vi "CheckOnIdle.vi"(6 "DataMessageQueue":refnum<queue>, 7 "ClassQueue":refnum<queue>, 8 "error in (no error)":errorcluster, 9 "Timeout (5s)":dbl=5.0 min=0.0 max=10.0, 10 "ChangeOccured? (F)":bool, 11 "SensorBase in":refnum<class "SensorBase.lvclass">) -> (0 "Error Out":errorcluster, 2 "Wrote?":bool, 3 "SensorBase out":refnum<class "SensorBase.lvclass">)   [LabVIEW 2018, in "SensorPlugins.lvlib"]
doc: "This VI checks to see if the module's acquistion loop is in idle. If it is it updates the Class Typedefinition that is stored in the queue. If it is not it sends a message to place it in idle, checks again and then updates the type definition if it is."
uses:
  SensorPlugins.lvlib
  SensorBaseClass/SensorBase.lvclass
  clMessage.ctl
  CheckOnIdle.ctl
  <vilib>/Utility/error.llb/Error Cluster From Error Code.vi
  <vilib>/ErrorRing/Error Ring.xnode
panel:
  out "Restart":bool
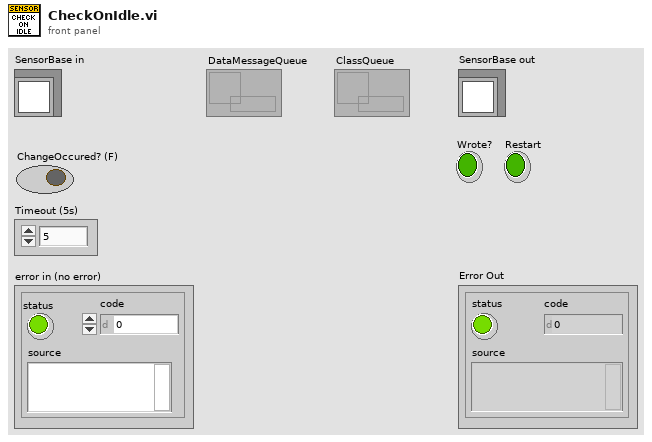
[diagram p1: front panel]
types:
  T1 = typedef "SensorPlugins.lvlib/CheckOnIdle.ctl" = enum16{"CheckOnState", "WriteToClassAndExit", "InIdle", "SetToStop", "Error", "Exit", "ReturnToStart"}
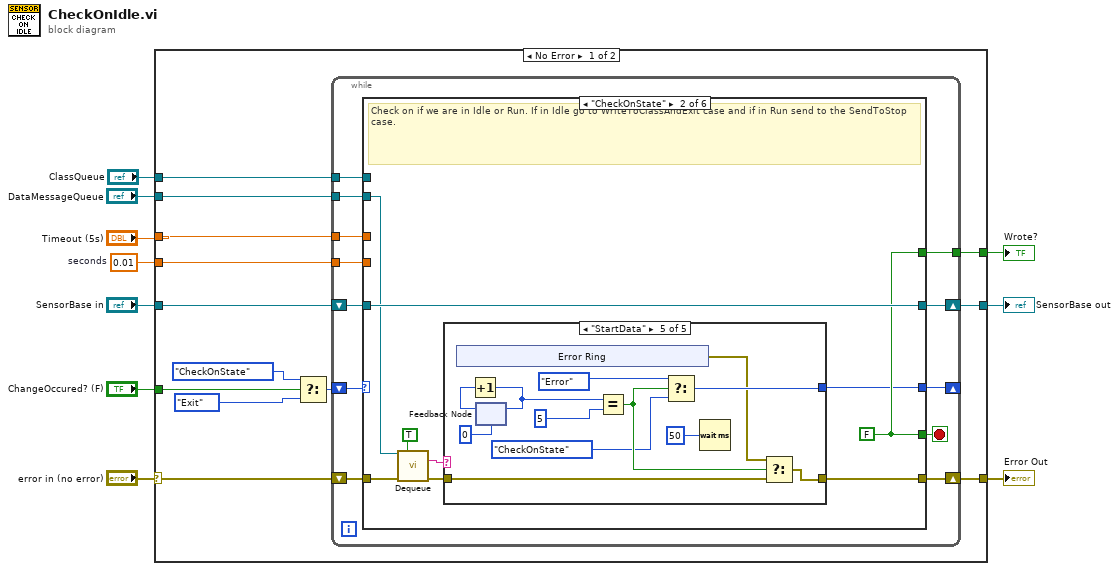
[diagram p0: block diagram]
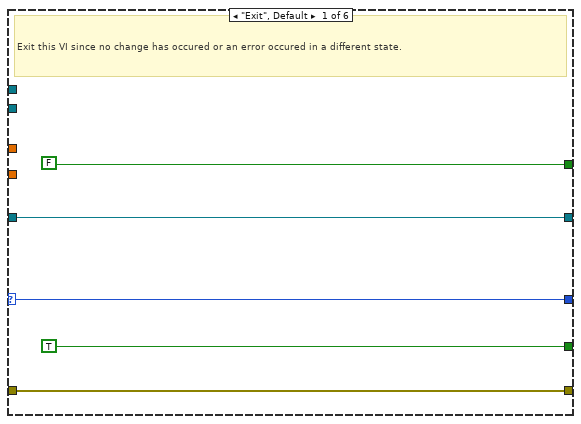
[diagram p2: hidden frame]
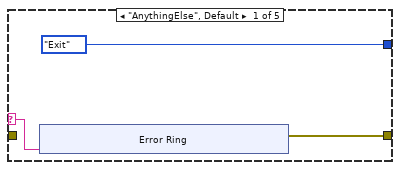
[diagram p3: hidden frame]
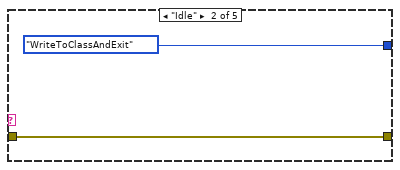
[diagram p4: hidden frame]
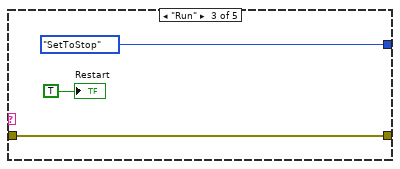
[diagram p5: hidden frame]
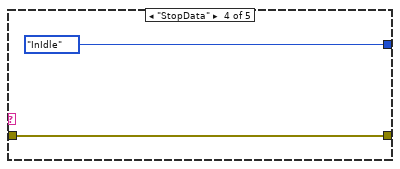
[diagram p6: hidden frame]
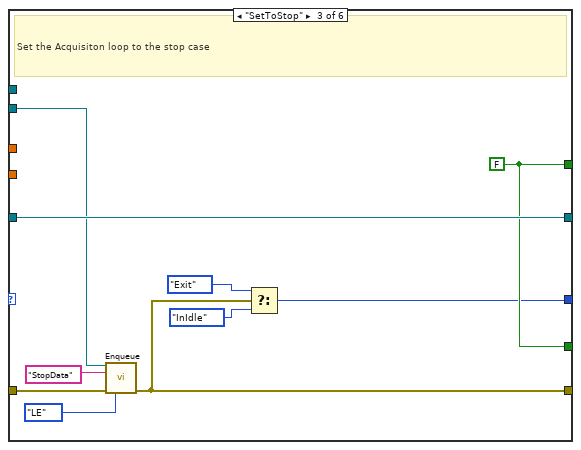
[diagram p7: hidden frame]
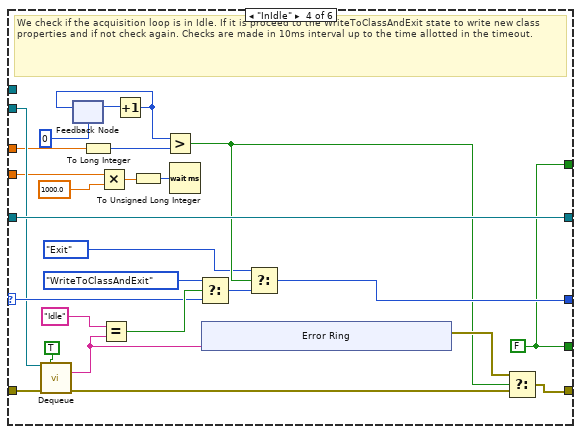
[diagram p8: hidden frame]
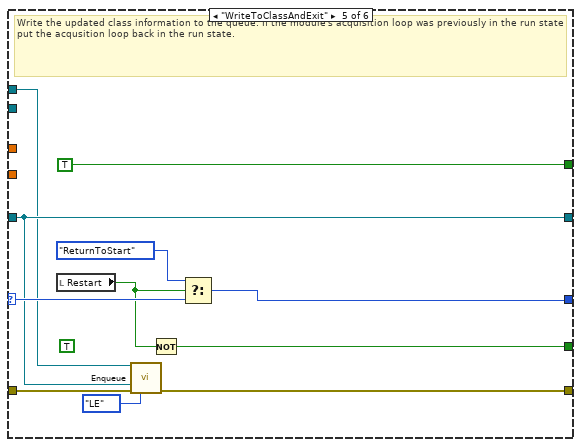
[diagram p9: hidden frame]
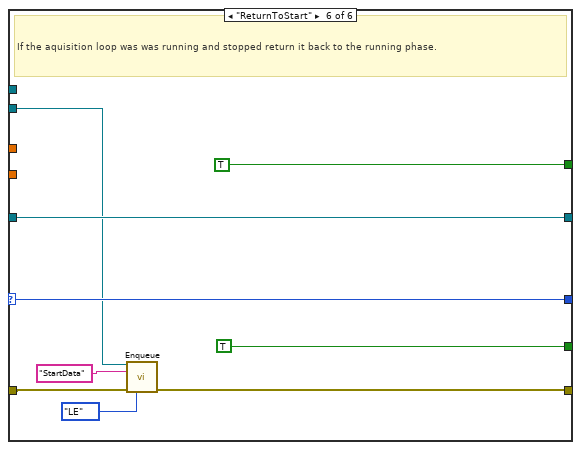
[diagram p10: hidden frame]
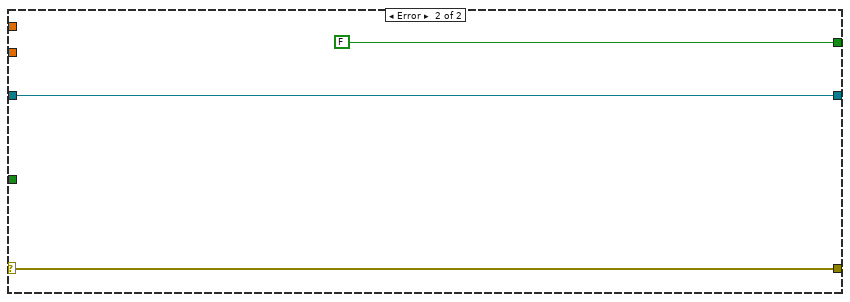
[diagram p11: hidden frame]
diagram:
  w9 = 0.01  # seconds
  n1 = case shown="No Error" "error in (no error)" {
    selector: "error in (no error)" -> [w22 w149]
    tunnel: "ChangeOccured? (F)" -> [w21 _]
    tunnel: "SensorBase in" -> [w20 w148]
    tunnel: [w19 w149] -> w6
    tunnel: "Timeout (5s)" -> [w18 _]
    tunnel: [w17 w148] -> w3
    tunnel: [w16 FALSE ("Set? (f)")] -> w5
    tunnel: "DataMessageQueue" -> [w15 _]
    tunnel: w9 -> [w14 _]
    tunnel: "ClassQueue" -> [w11 _]
    frame No Error {
      n2 = Select(t=CheckOnIdle."CheckOnState" ("Enum"), s=w21, f=CheckOnIdle."Exit" ("Enum")) -> (s? t:f=w23:T1)
      n3 = while {
        shift-right: [w30] -> _
        shift-left: w23 -> [w35]
        shift-right: [w32] -> w17
        shift-left: w20 -> [w33]
        shift-right: [w31] -> w19
        shift-left: w22 -> [w34]
        tunnel: w18 -> [w28]
        tunnel: [w27] -> w16
        tunnel: w15 -> [w26]
        tunnel: w14 -> [w25]
        tunnel: w11 -> [w24]
        stop <- w29 stop-if-true
        n4 = case shown="\"CheckOnState\"" w35 {
          selector: w35 -> [w39 _ _ w118 w134 w145]
          tunnel: w34 -> [w40 w48 w91 w111 w137 w140]
          tunnel: w33 -> [w38 w49 w93 w117 w128 w143]
          tunnel: [w40 w41 w88 w102 w130 w139] -> w31
          tunnel: [w38 w49 w93 w117 w128 w143] -> w32
          tunnel: [w39 w43 w87 w112 w135 w145] -> w30
          tunnel: [TRUE w45 w92 w104 w131 TRUE] -> w29
          tunnel: w28 -> [_ _ _ w96 _ _]
          tunnel: [FALSE ("Set? (f)") w45 w92 w104 TRUE ("Set? (f)") TRUE ("Set? (f)")] -> w27
          tunnel: w26 -> [_ w47 w90 w110 _ w138]
          tunnel: w25 -> [_ _ _ w106 _ _]
          tunnel: w24 -> [_ _ _ _ w127 _]
          frame "Exit", Default {
            # "Exit this VI since no change has occured or an error occured in a different state."
          }
          frame "CheckOnState" {
            w45 = FALSE
            # "Check on if we are in Idle or Run. If in Idle go to WriteToClassAndExit case and if in Run send to the SendToStop case."
            n5 = call "Dequeue.vi"("MessageQueue"=w47, "Preview Queue (F)"=TRUE ("PreviewQueue(F)"), "error in (no error)"=w48) -> ("Message"=w44:string, "error out"=w42:errorcluster)  [unwired: 8 in, 3 out]
            n6 = case shown="\"StartData\"" w44 {
              selector: w44 -> [w51 _ _ _ _]
              tunnel: [CheckOnIdle."Exit" ("Enum") CheckOnIdle."WriteToClassAndExit" ("Enum") CheckOnIdle."SetToStop" ("Enum") CheckOnIdle."InIdle" ("Enum") w76] -> w43
              tunnel: w42 -> [_ w61 w64 w66 w75]
              tunnel: [w52 w61 w64 w66 w74] -> w41
              frame "AnythingElse", Default {
                n7 = xnode "Error Ring"("parameter 0"=w51) -> ("error out"=w52:errorcluster)
              }
              frame "Idle" {
              }
              frame "Run" {
                "Restart" <- TRUE ("Restart")
              }
              frame "StopData" {
              }
              frame "StartData" {
                n8 = xnode "Error Ring"() -> ("error out"=w70:errorcluster)
                n9 = feedback #1(0) -> (w77:i32)
                n10 = Increment(x=w77) -> (x+1=w73:i32)
                n11 = feedback-in #1(w73) -> ()
                n12 = Equal?(x=w73, y=5 ("x")) -> (x = y?=w71:bool)
                n13 = Select(t=CheckOnIdle."Error" ("Enum"), s=w71, f=CheckOnIdle."CheckOnState" ("Enum")) -> (s? t:f=w76:T1)
                n14 = Wait (ms)(milliseconds to wait=u32 50) -> ()  [unwired: 1 out]
                n15 = Select(t=w70, s=w71, f=w75) -> (s? t:f=w74:errorcluster)
              }
            }
          }
          frame "SetToStop" {
            w92 = FALSE
            # "Set the Acquisiton loop to the stop case"
            n16 = call "Enqueue.vi"("MessageQueue"=w90, "Message"="StopData", "error in (no error)"=w91, "Type of Enqueue"=enum16{"Else", "LE"}."LE" ("Enum")) -> ("error out"=w88:errorcluster)  [unwired: 10 in, 1 out]
            n17 = Select(t=CheckOnIdle."Exit" ("Enum"), s=w88, f=CheckOnIdle."InIdle" ("Enum")) -> (s? t:f=w87:T1)
          }
          frame "InIdle" {
            w104 = FALSE
            # "We check if the acquisition loop is in Idle. If it is proceed to the WriteToClassAndExit state to write new class properties and if not check again. Checks are made in 10ms interval up to the time allotted in the timeout."
            n18 = call "Dequeue.vi"("MessageQueue"=w110, "Preview Queue (F)"=TRUE ("PreviewQueue(F)"), "error in (no error)"=w111) -> ("Message"=w99:string, "error out"=w98:errorcluster)  [unwired: 8 in, 3 out]
            n19 = feedback #2(0) -> (w115:i32)
            n20 = To Long Integer(number=w96) -> (32bit integer=w97:i32)
            n21 = Multiply(x=w106, y=1000.0) -> (x*y=w105:dbl)
            n22 = Equal?(x="Idle" ("State In"), y=w99) -> (x = y?=w119:bool)
            n23 = Increment(x=w115) -> (x+1=w114:i32)
            n24 = feedback-in #2(w114) -> ()
            n25 = To Unsigned Long Integer(number=w105) -> (unsigned 32bit integer=w108:u32)
            n26 = Greater?(x=w114, y=w97) -> (0:w101:bool)
            n27 = Wait (ms)(milliseconds to wait=w108) -> ()  [unwired: 1 out]
            n28 = Select(t=CheckOnIdle."WriteToClassAndExit" ("Enum"), s=w119, f=w118) -> (s? t:f=w113:T1)
            n29 = xnode "Error Ring"("parameter 0"=w99) -> ("error out"=w103:errorcluster)
            n30 = Select(t=CheckOnIdle."Exit" ("Enum"), s=w101, f=w113) -> (s? t:f=w112:T1)
            n31 = Select(t=w103, s=w101, f=w98) -> (s? t:f=w102:errorcluster)
          }
          frame "WriteToClassAndExit" {
            (unwired) TRUE
            # "Write the updated class information to the queue. If the module's acquisition loop was previously in the run state put the acqusition loop back in the run state."
            n32 = local read "Restart"() -> (w132:bool)
            n33 = call "Enqueue.vi"("MessageQueue"=w127, "SensorBase in"=w128, "error in (no error)"=w137, "Type of Enqueue"=enum16{"Else", "LE"}."LE") -> ("error out"=w130:errorcluster)  [unwired: 10 in, 1 out]
            n34 = Not(x=w132) -> (.not. x?=w131:bool)
            n35 = Select(t=CheckOnIdle."ReturnToStart", s=w132, f=w134) -> (s? t:f=w135:T1)
          }
          frame "ReturnToStart" {
            # "If the aquisition loop was was running and stopped return it back to the running phase."
            n36 = call "Enqueue.vi"("MessageQueue"=w138, "Message"="StartData", "error in (no error)"=w140, "Type of Enqueue"=enum16{"Else", "LE"}."LE" ("Enum")) -> ("error out"=w139:errorcluster)  [unwired: 10 in, 1 out]
          }
        }
      }
    }
    frame Error {
    }
  }
  "Error Out" <- w6
  "Wrote?" <- w5
  "SensorBase out" <- w3
